vi "Data_Read_Signal_From_Disk.vi"(8 "error in (no error)":errorcluster, 9 "filename":string, 10 "path":path, 11 "wfm info":T1) -> (0 "error out":errorcluster, 2 "data":i16[](array[numeric]), 3 "Size":i32, 5 "wfm info":T1)   [LabVIEW 2020]
doc: "This VI reads a raw dataset from a disk file with the following format :\n- number of points = one value (I32)\n- data = number of points * values (I16)\n- 1/sample rate, i.e. time step = one value (SGL or F32)\n- vertical range = one value (SGL)\n- offset = one value (SGL)\nCalibrated data are obtained with : data * vertical range + offset"
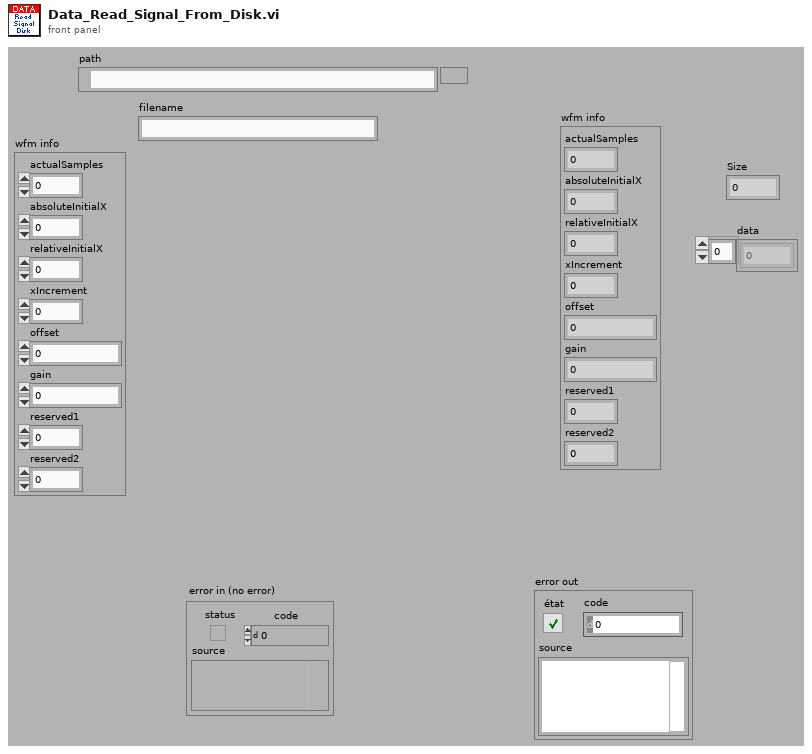
[diagram p1: front panel]
types:
  T1 = cluster{"actualSamples":i32, "absoluteInitialX":dbl, "relativeInitialX":dbl, "xIncrement":dbl, "offset":dbl, "gain":dbl, "reserved1":dbl, "reserved2":dbl}
  T2 = enum16{"big-endian, network order", "native, host order", "little-endian"}
  T3 = enum16{"open", "replace", "create", "open or create", "replace or create", "replace or create with confirmation"}
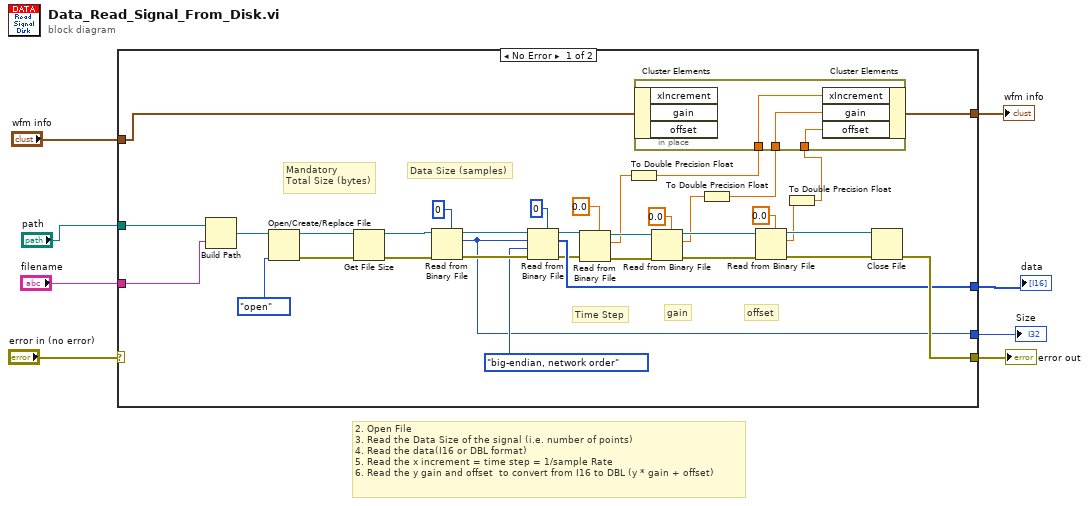
[diagram p0: block diagram]
diagram:
  # "2. Open File\n3. Read the Data Size of the signal (i.e. number of points)\n4. Read the data(I16 or DBL format)\n5. Read the x increment = time step = 1/sample Rate\n6. Read the y gain and offset  to convert from I16 to DBL (y * gain + offset)"
  n1 = case shown="No Error" "error in (no error)" {
    selector: "error in (no error)" -> [_ w48]
    tunnel: [w43 w48] -> w6
    tunnel: "wfm info" -> [w18 w47]
    tunnel: "path" -> [w40 _]
    tunnel: "filename" -> [w39 _]
    tunnel: [w30 _] -> w2
    tunnel: [w15 w47] -> w3
    tunnel: [w9 _] -> w1
    frame No Error {
      # "offset"
      # "gain"
      # "Time Step"
      # "Data Size (samples)"
      # "Mandatory\nTotal Size (bytes)"
      n2 = Build Path(base path=w40, name or relative path=w39) -> (appended path=w41:path)
      n3 = Open/Create/Replace File(file path (use dialog)=w41, operation (0:open)=T3."open" ("opération (0 : open)")) -> (refnum out=w32:refnum<file>, error out=w31:errorcluster)  [unwired: 4 in, 1 out]
      n4 = Get File Size(file=w32, error in=w31) -> (refnum out=w37:refnum<file>, 0:w36:errorcluster)  [unwired: 1 out]
      n5 = Read from Binary File(5:0, 8:w36, 11:w37) -> (0:w34:errorcluster, 2:w9:i32, 3:w35:refnum<file>)  [unwired: 3 in, 1 out]
      n6 = Read from Binary File(5:i16 0, 8:w34, 9:T2."big-endian, network order" ("ordre des octets (0 : big-Endian, network order)"), 10:w9, 11:w35) -> (0:w23:errorcluster, 2:w30:i16[], 3:w22:refnum<file>)  [unwired: 1 in, 1 out]
      n7 = Read from Binary File(5:sgl 0.0 ("type de données"), 8:w23, 11:w22) -> (0:w28:errorcluster, 2:w13:sgl, 3:w14:refnum<file>)  [unwired: 3 in, 1 out]
      n8 = To Double Precision Float(number=w13) -> (double precision float=w12:dbl)
      n9 = Read from Binary File(5:sgl 0.0 ("type de données"), 8:w28, 11:w14) -> (0:w25:errorcluster, 2:w16:sgl, 3:w26:refnum<file>)  [unwired: 3 in, 1 out]
      n10 = To Double Precision Float(number=w16) -> (double precision float=w11:dbl)
      n11 = Read from Binary File(5:sgl 0.0, 8:w25, 11:w26) -> (0:w20:errorcluster, 2:w17:sgl, 3:w21:refnum<file>)  [unwired: 3 in, 1 out]
      n12 = To Double Precision Float(number=w17) -> (double precision float=w10:dbl)
      n13 = in-place {
        in-place-border: w10 -> [w46]
        in-place-border: w11 -> [w45]
        in-place-border: w12 -> [w44]
        n14 = in-place-cluster #1(w18) -> ()  [unwired: 3 out]
        n15 = in-place-cluster #1("xIncrement"=w44, "gain"=w45, "offset"=w46) -> (w15:T1)
      }
      n16 = Close File(refnum=w21, error in=w20) -> (error out=w43:errorcluster)  [unwired: 1 out]
    }
    frame Error {
    }
  }
  "error out" <- w6
  "data" <- w2
  "wfm info" <- w3
  "Size" <- w1
